vi "SendCmd.vi"(8 "error in (no error)":errorcluster, 10 "cmd":string, 11 "FTP in":refnum<class "FTP.lvclass">) -> (0 "error out":errorcluster, 3 "FTP out":refnum<class "FTP.lvclass">)   [LabVIEW 2013, in "FTP.lvlib" / "FTP.lvclass"]
uses:
  FTP.lvclass
  controls/CmdCluster.ctl
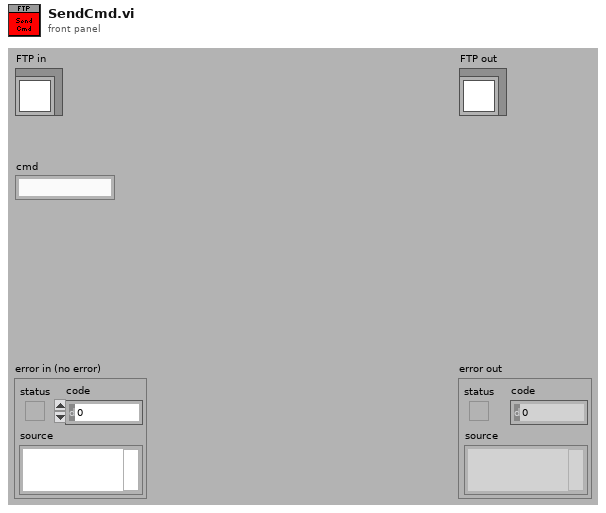
[diagram p1: front panel]
types:
  T1 = typedef "FTP.lvlib/FTP.lvclass/CmdCluster.ctl" = cluster{"CmdSting":string, "FromClient":bool}
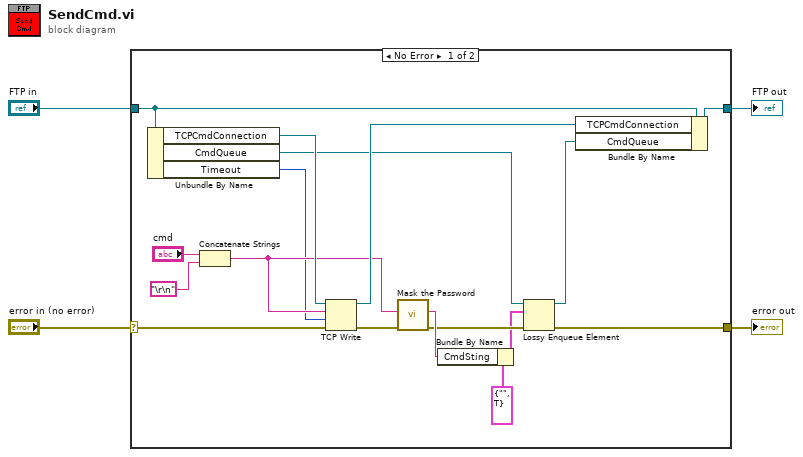
[diagram p0: block diagram]
diagram:
  n1 = case shown="No Error" "error in (no error)" {
    selector: "error in (no error)" -> [w7 w23]
    tunnel: [w15 w23] -> w3
    tunnel: [w19 w22] -> w1
    tunnel: "FTP in" -> [w21 w22]
    frame No Error {
      n2 = Unbundle By Name(w21) -> ("TCPCmdConnection"=w20:refnum<k5>, "CmdQueue"=w14:refnum<queue>, "Timeout"=w6:i32)
      n3 = Concatenate Strings("cmd", "\r\n") -> (w11:string)
      n4 = TCP Write(connection ID=w20, data in=w11, error in (no error)=w7, 9:w6) -> (connection ID out=w18:refnum<k5>, error out=w9:errorcluster)  [unwired: 1 out]
      n5 = call "Mask the Password.vi"("error in (no error)"=w9, "Cmd String in"=w11) -> ("error out"=w8:errorcluster, "Cmd String out"=w10:string)  [unwired: 8 in]
      n6 = Bundle By Name(cluster=T1 {"CmdSting"="", "FromClient"=TRUE} ("CmdCluster"), "CmdSting"=w10) -> (w5:T1)
      n7 = Lossy Enqueue Element(queue=w14, element=w5, error in (no error)=w8) -> (queue out=w13:refnum<queue>, error out=w15:errorcluster)  [unwired: 2 out]
      n8 = Bundle By Name(cluster=w21, "TCPCmdConnection"=w18, "CmdQueue"=w13) -> (w19:refnum<class "FTP.lvclass">)
    }
    frame Error {
    }
  }
  "error out" <- w3
  "FTP out" <- w1
